vi "Prepare measurement.vi"(7 "Instr info":T2 {"PwrMonitor"."Last update" format="%<%H:%M:%S>T"; "VTI"."Last update" format="%<%H:%M:%S>T"; "PMD"."Last update" format="%<%H:%M:%S>T"; "SMU"."Last update" format="%<%H:%M:%S>T"; "Servo"."Last update" format="%<%H:%M:%S>T"; "Rotator"."Actuator" items=["Linear", "Roatator", "Goniometer"]; "Rotator"."Name" items=["ANC350res", "ANC350num", "ANC350fps", "Unknown"]; "Rotator"."Last update" format="%<%H:%M:%S>T"; "THz"."Last update" format="%<%H:%M:%S>T"; "MFLI"."Last update" format="%<%H:%M:%S>T"; "Magnet"."Last update" format="%<%H:%M:%S>T"}, 9 "VID control":T1={"AMC"=9, "Multip"=1, "Base frequency [GHz]"=0.0, "End frequency [GHz]"=0.0, "Im frequency [MHz]"=1500.0, "Sweep up [ms]"=0.0, "Reset trigger?"=FALSE} {"Multip" items=["1"=1, "2"=2, "3"=3, "4"=4, "6"=6, "8"=8, "9"=9]; "AMC" items=["9"=9, "12"=12]; "End frequency [GHz]" min=0.00018 max=20000.0; "Base frequency [GHz]" min=81.0 max=126.0 format="%.2g"}, 10 "Script cluster":T6={"Start"=nan, "Start Caption"="Start [T]", "End"=0.0, "End Caption"="End [T]", "Sweep"=0.0, "Sweep caption"="Rate [mT/s]", "Constant"=0.0, "Constant caption"="Freq [GHz]", "Mod_F [kHz]"=0.0, "Mod_A [G]"=0.0, "Tau [ms]"=0.0, "Angle [°]"=0.0, "Tmp [K]"=50.0, "Wait [min]"=0.0, "Carousel"=-1, "Comment"="", "Auto-mod"=TRUE, "Execute"=FALSE} {"Carousel" items=["0", "1", "2", "3", "4", "5", "6"]; "Angle [°]" min=0.0 max=350.0; "Tau [ms]" min=0.0 max=100.0; "Wait [min]" min=0.0 max=350.0; "Tmp [K]" min=0.0 max=3000.0; "Mod_A [G]" min=0.1 max=150.0; "Mod_F [kHz]" min=0.1 max=150.0}, 11 "Referencies in":T7) -> (0 "error out":errorcluster)   [LabVIEW 2024]
uses:
  Subsystem modules/Messenger service/Data types/Messenger referencies.ctl
  Datatypes/script polymorh line.ctl
  Datatypes/Instr Info.ctl
  Subsystem modules/Magnet module/ctl/RampingOutput.ctl
  Datatypes/Single servo status.ctl
  Subsystem modules/Servo drive module/ctl/Axis names.ctl
  Datatypes/THz parameters.ctl
  Subsystem modules/Magnet module/ctl/MSG to magnet.ctl
  Subsystem modules/Magnet module/ctl/Magnet Orders.ctl
  Subsystem modules/Magnet module/ctl/SetField data.ctl
  Subsystem modules/Magnet module/ctl/Magnet mode public.ctl
  Subsystem modules/Lock-in module/ctl/MFLI_message for module.ctl
  Subsystem modules/Lock-in module/ctl/MFLI_command enum.ctl
  Subsystem modules/Lock-in module/ctl/MFLI_parameter and value.ctl
  Subsystem modules/Lock-in module/ctl/MFLI_node.ctl
  Subsystem modules/THz module/ctl/THz sweep parameters.ctl
  Subsystem modules/Temperature control module/ctl/MSG for VTI.ctl
  Subsystem modules/Temperature control module/ctl/TC commands.ctl
  Subsystem modules/THz module/ctl/THz Message for module.ctl
  Subsystem modules/THz module/ctl/THz commands enum.ctl
  Subsystem modules/Temperature control module/ctl/Set point.ctl
  Subsystem modules/Sample rotator/ctl/MSG to Rotator.ctl
  Subsystem modules/Sample rotator/ctl/Rotator commands.ctl
  Subsystem modules/Sample rotator/ctl/Positoin to set.ctl
  Subsystem modules/Magnet module/Magnet module.lvlib
  Subsystem modules/THz module/THz source modeule.lvlib
  Subsystem modules/Lock-in module/Lock-in module.lvlib
  Subsystem modules/Temperature control module/Temperature controller.lvlib
  Subsystem modules/Sample rotator/SampleRotator.lvlib
  Subsystem modules/Messenger service/MessengerLib.lvlib
  Subsystem modules/Servo drive module/Servo drive module.lvlib
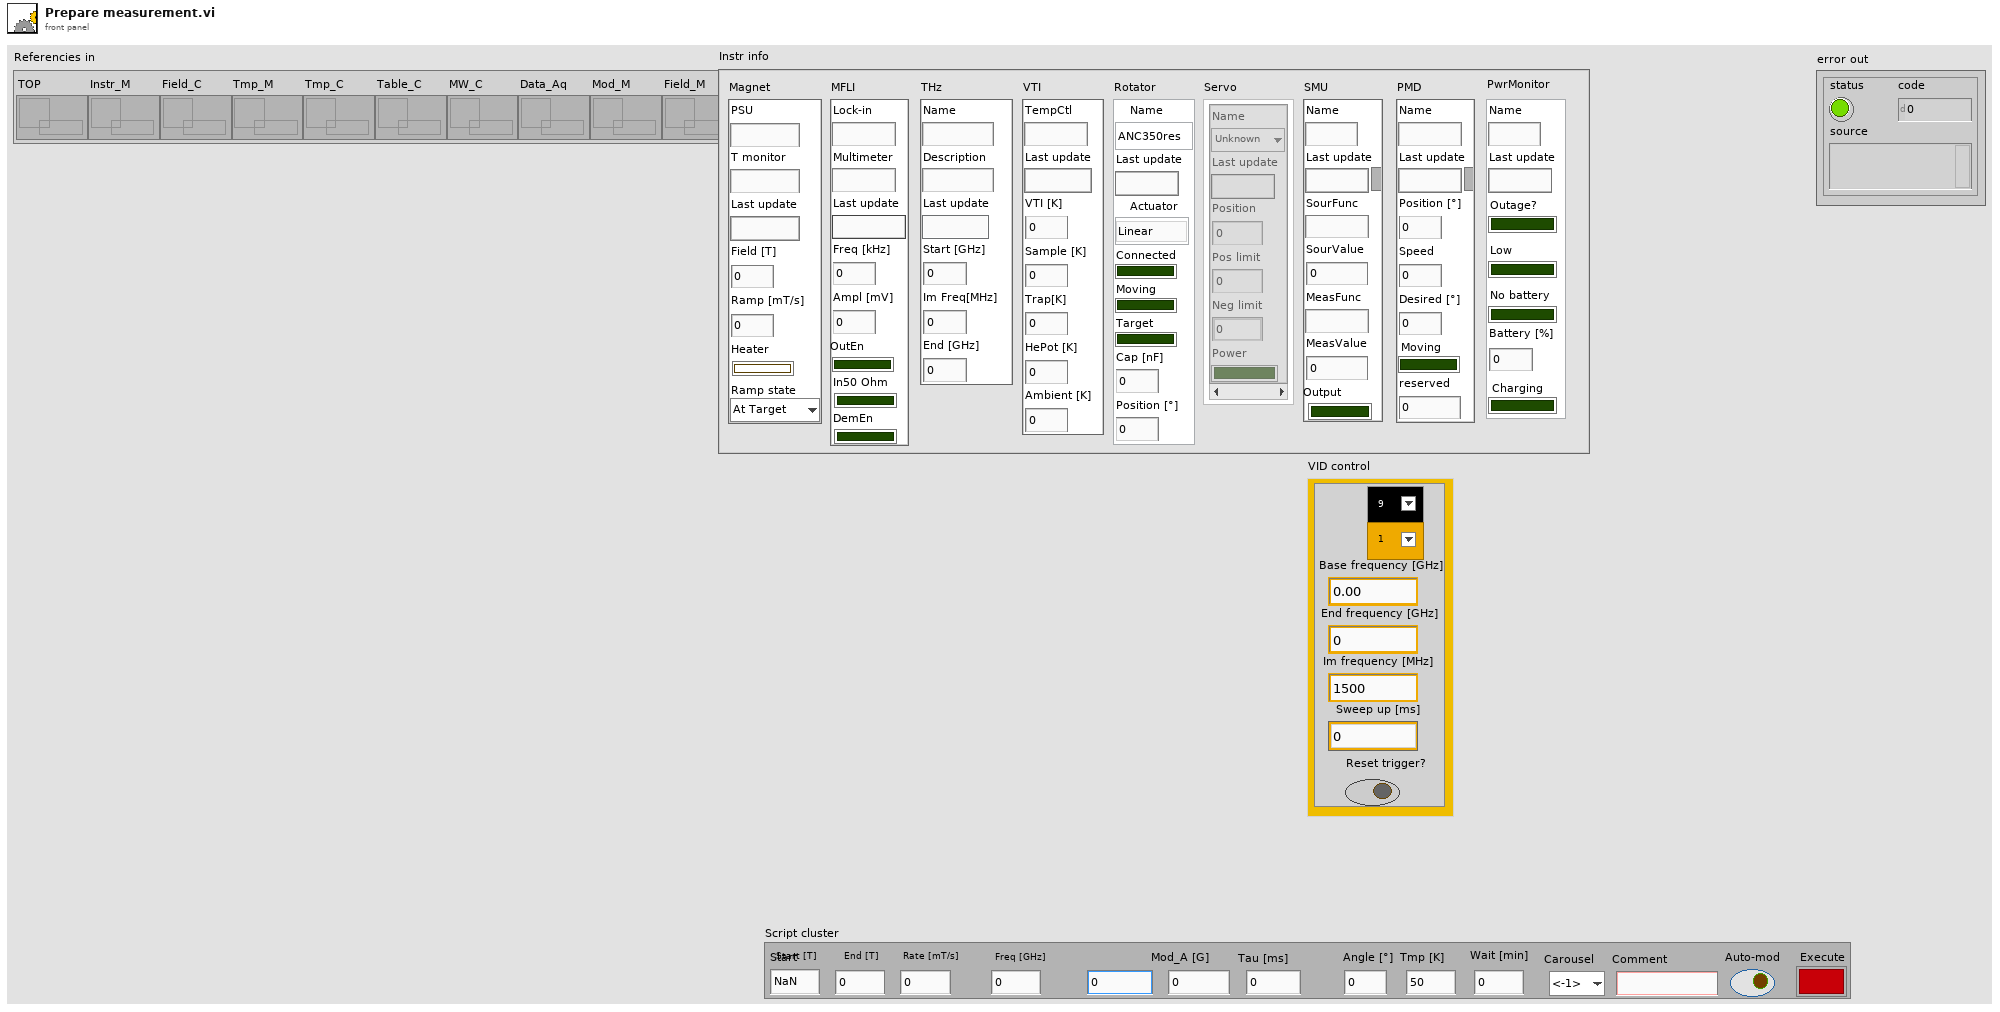
[diagram p1: front panel]
types:
  T1 = typedef "THz parameters.ctl" = cluster{"AMC":u16, "Multip":u16, "Base frequency [GHz]":dbl, "End frequency [GHz]":dbl, "Im frequency [MHz]":dbl, "Sweep up [ms]":dbl, "Reset trigger?":bool}
  T2 = typedef "Instr Info.ctl" = cluster{"Magnet":cluster{"PSU":string, "T monitor":string, "Last update":timestamp, "Field [T]":dbl, "Ramp [mT/s]":dbl, "Heater":bool, "Ramp state":T3}, "MFLI":cluster{"Lock-in":string, "Multimeter":string, "Last update":timestamp, "Freq [kHz]":dbl, "Ampl [mV]":dbl, "OutEn":bool, "In50 Ohm":bool, "DemEn":bool}, "THz":cluster{"Name":string, "Description":string, "Last update":timestamp, "Start [GHz]":dbl, "Im Freq[MHz]":dbl, "End [GHz]":dbl}, "VTI":cluster{"TempCtl":string, "Last update":timestamp, "VTI [K]":dbl, "Sample [K]":dbl, "Trap[K]":dbl, "HePot [K]":dbl, "Ambient [K]":dbl}, "Rotator":cluster{"Name":u16, "Last update":timestamp, "Actuator":u16, "Connected":bool, "Moving":bool, "Target":bool, "Cap [nF]":dbl, "Position [°]":dbl}, "Servo":T4[], "SMU":cluster{"Name":string, "Last update":timestamp, "SourFunc":string, "SourValue":dbl, "MeasFunc":string, "MeasValue":dbl, "Output":bool}, "PMD":cluster{"Name":string, "Last update":timestamp, "Position [°]":dbl, "Speed":dbl, "Desired [°]":dbl, "Moving":bool, "reserved":dbl}, "PwrMonitor":cluster{"Name":string, "Last update":timestamp, "Outage?":bool, "Low":bool, "No battery":bool, "Battery [%]":u8, "Charging":bool}}
  T3 = typedef "Magnet module.lvlib/RampingOutput.ctl" = enum16{"At Target", "Go up", "Go down"}
  T4 = typedef "Single servo status.ctl" = cluster{"Name":T5, "Last update":timestamp, "Position":dbl, "Pos limit":dbl, "Neg limit":dbl, "Power":bool}
  T5 = typedef "Servo drive module.lvlib/Axis names.ctl" = enum16{"Unknown", "AxisX", "AxisY", "AxisZ_left", "AxisZ_middle", "AxisZ_right"}
  T6 = typedef "script polymorh line.ctl" = cluster{"Start":dbl, "Start Caption":string, "End":dbl, "End Caption":string, "Sweep":dbl, "Sweep caption":string, "Constant":dbl, "Constant caption":string, "Mod_F [kHz]":dbl, "Mod_A [G]":dbl, "Tau [ms]":dbl, "Angle [°]":dbl, "Tmp [K]":dbl, "Wait [min]":dbl, "Carousel":i8, "Comment":string, "Auto-mod":bool, "Execute":bool}
  T7 = typedef "MessengerLib.lvlib/Messenger referencies.ctl" = cluster{"TOP":refnum<queue>, "Instr_M":refnum<queue>, "Field_C":refnum<queue>, "Tmp_M":refnum<queue>, "Tmp_C":refnum<queue>, "Table_C":refnum<queue>, "MW_C":refnum<queue>, "Data_Aq":refnum<queue>, "Mod_M":refnum<queue>, "Field_M":refnum<queue>, "Pwr_M":refnum<queue>, "Angle_C":refnum<queue>, "Sample_C":refnum<queue>, "Reserved":refnum<queue>}
  T8 = typedef "Lock-in module.lvlib/MFLI_parameter and value.ctl" = cluster{"parameter":T9, "value":dbl}
  T9 = typedef "Lock-in module.lvlib/MFLI_node.ctl" = enum16{"None", "filter_order [-]", "filter_constant [ms]", "in_diff", "in_autorange", "in_imp50", "in_AC", "osc_freq [kHz]", "out_ampl [V]", "out_autorange", "out_imp50", "enable output", "enamble ampl", "scope_enable", "scope_rate", "scope_len", "scope_trigEn", "AuxOut_amplify", "Phase_deg", "AuxOut_select"}
  T10 = typedef "Magnet module.lvlib/Magnet mode public.ctl" = enum16{"Persistant", "Ramping"}
  T11 = typedef "Magnet module.lvlib/MSG to magnet.ctl" = cluster{"Order":T12, "Data":variant}
  T12 = typedef "Magnet module.lvlib/Magnet Orders.ctl" = enum16{"Ignore", "Connect", "Update", "Switch mode", "Set field", "Stop ramping", "Equalize output", "Zero output", "Flip polarity", "Blackout", "Set timer", "Eval temperatures", "Disconnect"}
  T13 = typedef "Temperature controller.lvlib/Set point.ctl" = cluster{"Heater":string, "Tmp [K]":dbl}
  T14 = typedef "THz source modeule.lvlib/THz Message for module.ctl" = cluster{"Command":T15, "Data":variant}
  T15 = typedef "THz source modeule.lvlib/THz commands enum.ctl" = enum16{"Ignore", "Connect", "Update", "Set parameters", "Disconnect", "End"}
  T16 = typedef "Temperature controller.lvlib/MSG for VTI.ctl" = cluster{"Command":T17, "Data":variant}
  T17 = typedef "Temperature controller.lvlib/TC commands.ctl" = enum16{"Initialize", "Update", "Stop tmp change", "Set temperature", "Set point", "Disconnect", "End", "Ignore"}
  T18 = typedef "THz source modeule.lvlib/THz sweep parameters.ctl" = cluster{"Start [GHz]":dbl, "End [GHz] ":dbl, "Sweep up\ntime [ms]":dbl, "Sweep down\ntime [ms]":dbl, "Intermidiate [MHz]":dbl, "Reset trigger":bool}
  T19 = typedef "Lock-in module.lvlib/MFLI_message for module.ctl" = cluster{"Command":T20, "Data":variant}
  T20 = typedef "Lock-in module.lvlib/MFLI_command enum.ctl" = enum16{"Initialize", "Update", "Set parameters", "Set module", "Set individual parameters", "Get point", "Get array", "Disconnect", "End", "Ignore"}
  T21 = typedef "Magnet module.lvlib/SetField data.ctl" = cluster{"Field [T]":dbl, "Ramp [T/s]":dbl, "Custom Ramp?":bool, "Mode":T10}
  T22 = typedef "Positoin to set.ctl" = cluster{"Relative?":bool, "Position [°]":dbl, "Safe to move?":bool}
  T23 = typedef "SampleRotator.lvlib/MSG to Rotator.ctl" = cluster{"Command":T24, "Data":variant}
  T24 = typedef "SampleRotator.lvlib/Rotator commands.ctl" = enum16{"Ignore", "Initialize", "Update", "Set parameters", "Stop movement", "Set position", "Disconnect", "End"}
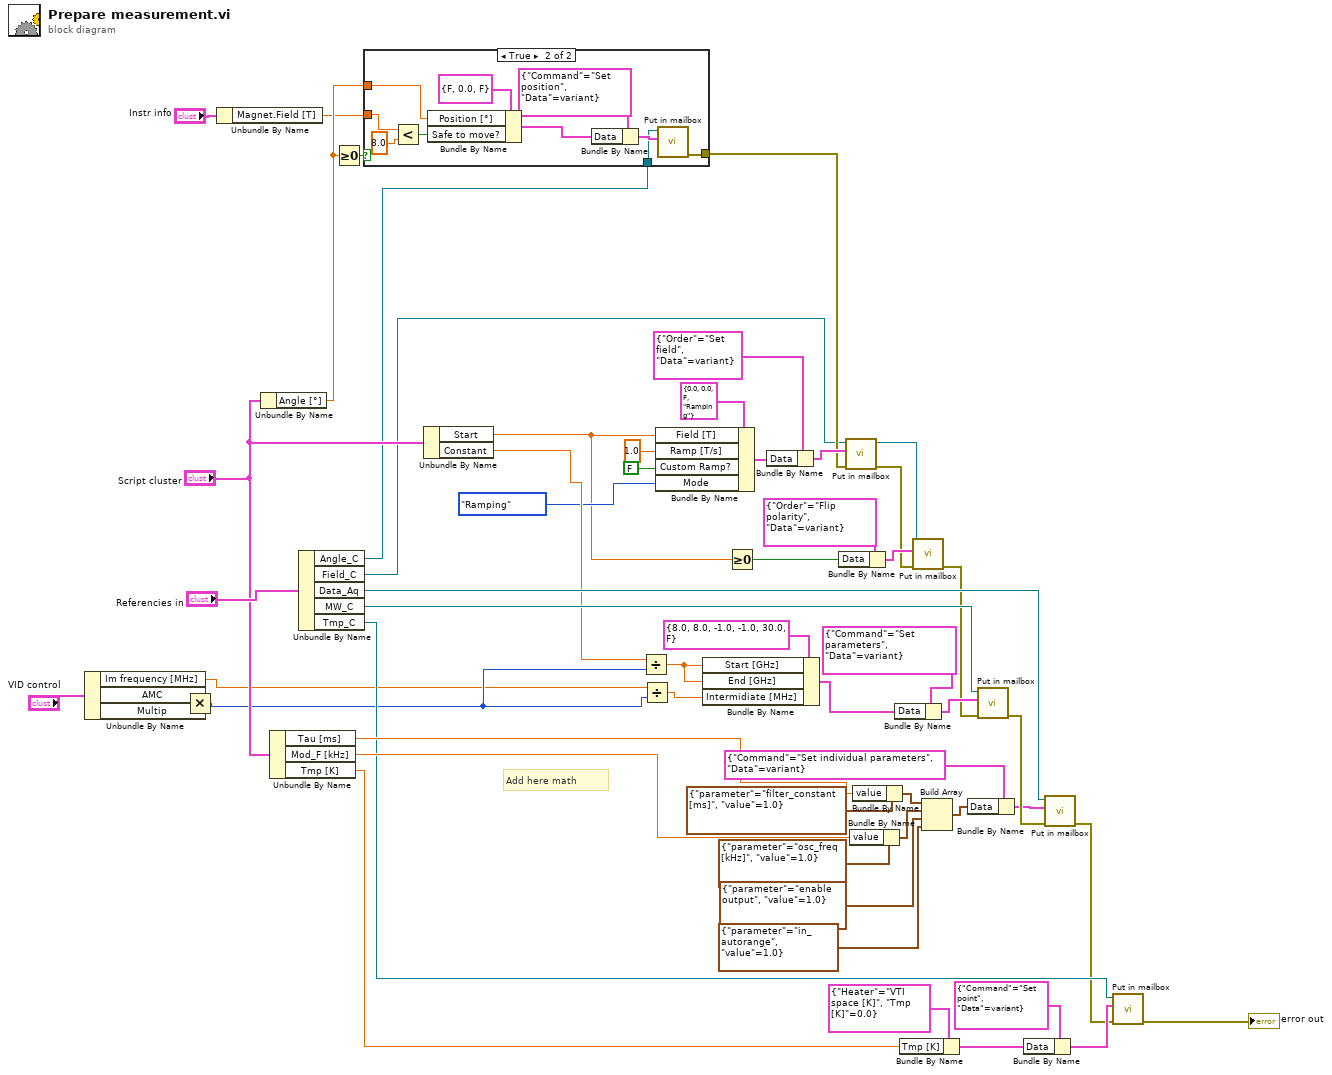
[diagram p0: block diagram]
diagram:
  # "Add here math"
  n1 = Unbundle By Name("VID control") -> ("Im frequency [MHz]"=w2:dbl, "AMC"=w5:u16, "Multip"=w4:u16)
  n2 = Multiply(x=w5, y=w4) -> (x*y=w3:u16)
  n3 = Unbundle By Name("Instr info") -> ("Magnet.Field [T]"=w17:dbl)
  n4 = Unbundle By Name("Script cluster") -> ("Angle [°]"=w19:dbl)
  n5 = Unbundle By Name("Script cluster") -> ("Tau [ms]"=w40:dbl, "Mod_F [kHz]"=w39:dbl, "Tmp [K]"=w7:dbl)
  n6 = Unbundle By Name("Referencies in") -> ("Angle_C"=w21:refnum<queue>, "Field_C"=w11:refnum<queue>, "Data_Aq"=w34:refnum<queue>, "MW_C"=w33:refnum<queue>, "Tmp_C"=w38:refnum<queue>)
  n7 = Greater Or Equal To 0?(x=w19) -> (x >= 0?=w20:bool)
  n8 = case shown="True" w20 {
    tunnel: [_ w62] -> w12
    tunnel: w21 -> [_ w61]
    tunnel: w19 -> [_ w60]
    tunnel: w17 -> [_ w59]
    frame False {
    }
    frame True {
      n9 = Less?(x=w59, y=8.0) -> (x < y?=w58:bool)
      n10 = Bundle By Name(cluster=T22 {"Relative?"=FALSE, "Position [°]"=0.0, "Safe to move?"=FALSE} ("Set position"), "Position [°]"=w60, "Safe to move?"=w58) -> (w63:T22)
      n11 = Bundle By Name(cluster=T23 {"Command"=enum."Set position", "Data"=variant} ("MSG to rotator"), "Data"=w63) -> (w64:T23)
      n12 = call "Put in mailbox.vi"("Message"=w64, "Queue in"=w61) -> ("error out"=w62:errorcluster)  [unwired: 7 in, 2 out]
    }
  }
  n13 = Unbundle By Name("Script cluster") -> ("Start"=w13:dbl, "Constant"=w23:dbl)
  n14 = Divide(x=w23, y=w3) -> (x/y=w41:dbl)
  n15 = Divide(x=w2, y=w3) -> (x/y=w29:dbl)
  n16 = Bundle By Name(cluster=T21 {"Field [T]"=0.0, "Ramp [T/s]"=0.0, "Custom Ramp?"=FALSE, "Mode"=enum."Ramping"} ("Set Field"), "Field [T]"=w13, "Ramp [T/s]"=1.0, "Custom Ramp?"=FALSE, "Mode"=Magnet_mode_public."Ramping") -> (w56:T21)
  n17 = Bundle By Name(cluster=T18 {"Start [GHz]"=8.0, "End [GHz] "=8.0, "Sweep up\ntime [ms]"=-1.0, "Sweep down\ntime [ms]"=-1.0, "Intermidiate [MHz]"=30.0, "Reset trigger"=FALSE} ("Sweep parameters"), "Start [GHz]"=w41, "End [GHz]"=w41, "Intermidiate [MHz]"=w29) -> (w31:T18)
  n18 = Greater Or Equal To 0?(x=w13) -> (x >= 0?=w14:bool)
  n19 = Bundle By Name(cluster=T11 {"Order"=enum."Set field", "Data"=variant} ("MSG to magnet"), "Data"=w56) -> (w57:T11)
  n20 = Bundle By Name(cluster=T11 {"Order"=enum."Flip polarity", "Data"=variant} ("MSG to magnet"), "Data"=w14) -> (w15:T11)
  n21 = call "Put in mailbox.vi"("error in (no error)"=w12, "Message"=w57, "Queue in"=w11) -> ("error out"=w9:errorcluster, "Queue out"=w8:refnum<queue>)  [unwired: 6 in, 1 out]
  n22 = Bundle By Name(cluster=T8 {"parameter"=enum."osc_freq [kHz]", "value"=1.0} ("Parameter to set"), "value"=w39) -> (w43:T8)
  n23 = Bundle By Name(cluster=T8 {"parameter"=enum."filter_constant [ms]", "value"=1.0} ("Parameter to set"), "value"=w40) -> (w46:T8)
  n24 = Bundle By Name(cluster=T14 {"Command"=enum."Set parameters", "Data"=variant} ("Incoming msg"), "Data"=w31) -> (w30:T14)
  n25 = Bundle By Name(cluster=T13 {"Heater"="VTI space [K]", "Tmp [K]"=0.0} ("Set point"), "Tmp [K]"=w7) -> (w25:T13)
  n26 = call "Put in mailbox.vi"("error in (no error)"=w9, "Message"=w15, "Queue in"=w8) -> ("error out"=w10:errorcluster)  [unwired: 6 in, 2 out]
  n27 = Build Array(w46, w43, T8 {"parameter"=enum."enable output", "value"=1.0} ("Parameter to set"), T8 {"parameter"=enum."in_autorange", "value"=1.0} ("Parameter to set")) -> (w44:T8[])
  n28 = Bundle By Name(cluster=T19 {"Command"=enum."Set individual parameters", "Data"=variant} ("MSG for  ACQ"), "Data"=w44) -> (w48:T19)
  n29 = call "Put in mailbox.vi"("error in (no error)"=w10, "Message"=w30, "Queue in"=w33) -> ("error out"=w52:errorcluster)  [unwired: 6 in, 2 out]
  n30 = Bundle By Name(cluster=T16 {"Command"=enum."Set point", "Data"=variant} ("MSG for VTI"), "Data"=w25) -> (w35:T16)
  n31 = call "Put in mailbox.vi"("error in (no error)"=w52, "Message"=w48, "Queue in"=w34) -> ("error out"=w27:errorcluster)  [unwired: 6 in, 2 out]
  n32 = call "Put in mailbox.vi"("error in (no error)"=w27, "Message"=w35, "Queue in"=w38) -> ("error out"=→"error out":errorcluster)  [unwired: 6 in, 2 out]
